vi "measure.vi"(8 "error in (no error)":errorcluster, 11 "DmmKeysight in":refnum<class "DmmKeysight.lvclass">) -> (0 "error out":errorcluster, 2 "value":dbl, 3 "DmmKeysight out":refnum<class "DmmKeysight.lvclass">)   [LabVIEW 2023, in "DmmKeysight.lvclass"]
doc: "<b>Author:</b> Wolfgang\n<b>Description:</b> initiate a measurement on Dmm and return result"
uses:
  DmmKeysight.lvclass
  DmmKeysight.lvclass/DmmKeysight.ctl
  Driver/Keysight-34450A.lvlib
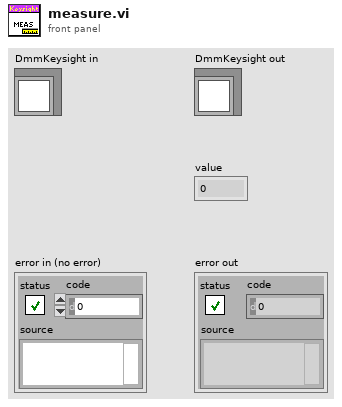
[diagram p1: front panel]
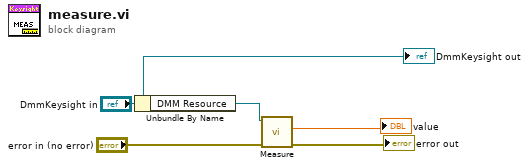
[diagram p0: block diagram]
diagram:
  n1 = Unbundle By Name("DmmKeysight in") -> ("DMM Resource"=w5:refnum<visa-resource-name>)
  n2 = call "Measure.vi"("error in (no error)"="error in (no error)", "VISA resource name"=w5) -> ("error out"=→"error out":errorcluster, "Measured Value"=→"value":dbl)  [unwired: 7 in, 1 out]
  "DmmKeysight out" <- "DmmKeysight in"
